vi "Shooter Immediate with Deadband.vi"(1 "POVs":bool, 2 "Shoot":bool, 3 "Reset":bool, 4 "Shot Position":dbl, 5 "Command Info In":T3, 6 "Auto-Shot":bool, 7 "Reset Values":T1, 8 "Setpoints":cluster{"Shooter":dbl, "Turret":dbl, "Hood":dbl}, 9 "Homing?":bool, 10 "Operation":T2) -> (0 "Command Info Out":T3)   [LabVIEW 2019]
doc: "This template includes code for deadband comparision to avoid excessive command scheduling. It is particularly useful for joystick-driven commands.\n\nBe sure to right-click and select New from Template and save with a new command name."
uses:
  <vilib>/Rock Robotics/WPI/Framework/Command Status Info.ctl
  <vilib>/Rock Robotics/WPI/Framework/Completion Status.ctl
  <vilib>/Rock Robotics/WPI/Framework/Completion Notifier.ctl
  Implementation/Shooter Operations.ctl
  Implementation/Shooter Setpoints.ctl
  Framework/Robot Global Data.vi
panel:
  in  "Description":string
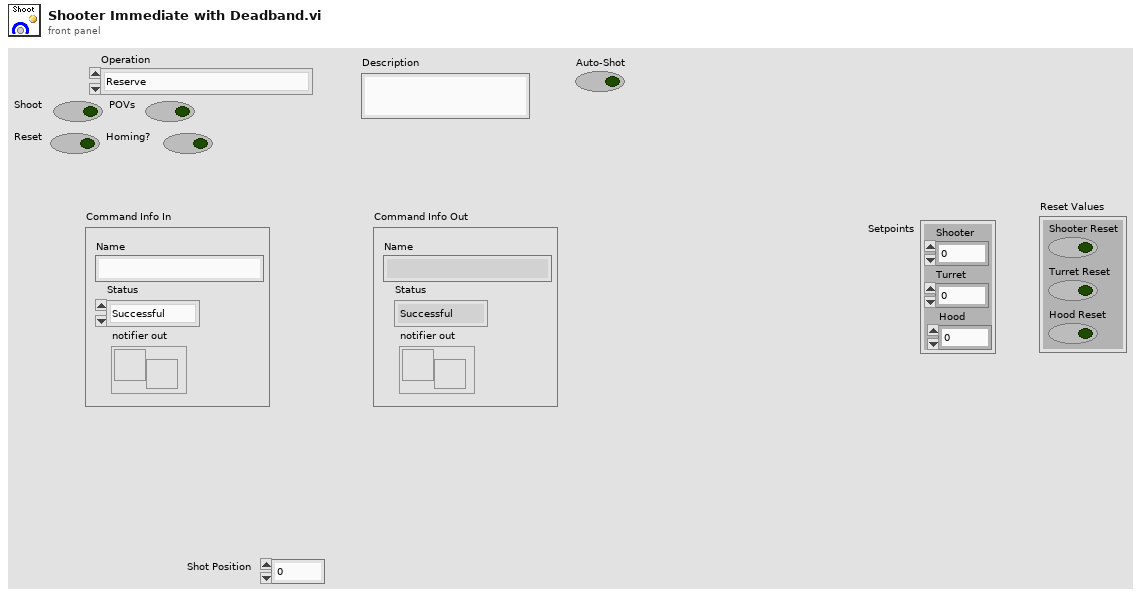
[diagram p1: front panel]
types:
  T1 = cluster{"Shooter Reset":bool, "Turret Reset":bool, "Hood Reset":bool}
  T2 = typedef "Shooter Operations.ctl" = enum16{"Reserve", "Read Current", "Immediate"}
  T3 = typedef "Command Status Info.ctl" = cluster{"Name":string, "Status":T4, "notifier out":T5}
  T4 = typedef "Completion Status.ctl" = enum16{"Successful", "Aborted", "Incomplete"}
  T5 = typedef "Completion Notifier.ctl" = refnum<notifier>
  T6 = typedef "Shooter Setpoints.ctl" = cluster{"Operation":T2, "Setpoints":cluster{"Shooter":dbl, "Turret":dbl, "Hood":dbl}, "Reset Values":cluster{"Shooter Reset":bool, "Turret Reset":bool, "Hood Reset":bool}, "Auto-Shot":bool, "Shoot":bool, "Reset":bool, "POVs":bool, "Homing?":bool}
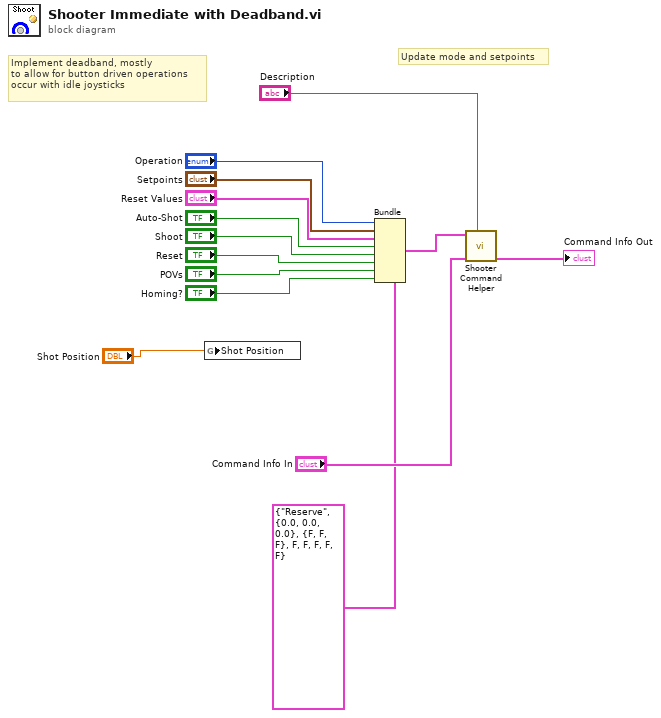
[diagram p0: block diagram]
diagram:
  # "Implement deadband, mostly\nto allow for button driven operations\noccur with idle joysticks"
  # "Update mode and setpoints"
  n1 = global write "Robot Global Data.vi" "Shot Position"("Shot Position") -> ()
  n2 = Bundle(cluster=T6 {"Operation"=enum."Reserve", "Setpoints"={"Shooter"=0.0, "Turret"=0.0, "Hood"=0.0}, "Reset Values"={"Shooter Reset"=FALSE, "Turret Reset"=FALSE, "Hood Reset"=FALSE}, "Auto-Shot"=FALSE, "Shoot"=FALSE, "Reset"=FALSE, "POVs"=FALSE, "Homing?"=FALSE} ("SubSystem Data"), "Operation"="Operation", "Setpoints"="Setpoints", "Reset Values"="Reset Values", "Auto-Shot"="Auto-Shot", "Shoot"="Shoot", "Reset"="Reset", "POVs"="POVs", "Homing?"="Homing?") -> (w9:T6)
  n3 = call "Shooter Command Helper.vi"("Description"="Description", "Command Info In"="Command Info In", "SubSystem Data"=w9) -> ("Command Info Out"=→"Command Info Out":T3)  [unwired: 6 in, 2 out]
